vi "test Get Attribute as JSON Array2.vi"(11 "Test Case In":refnum<class "Test Config From Excel Table.lvclass">) -> (0 "error out":errorcluster, 3 "Test Case Out":refnum<class "Test Config From Excel Table.lvclass">)   [LabVIEW 2020, in "Test Config From Excel Table.lvclass"]
uses:
  Test Config From Excel Table.lvclass
  Test Config From Excel Table.lvclass/Test Config From Excel Table.ctl
  <vilib>/JDP Science/JSONtext/JSONtext.lvlib
  <vilib>/Astemes/LUnit/Test Case.lvclass
  Open-Xml-LabVIEW/Source/Open Xml.lvlib
  Source/Config from Excel Table/Config from Excel Table.lvclass
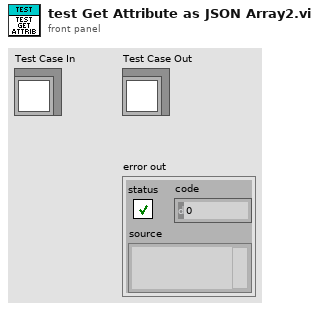
[diagram p1: front panel]
types:
  T1 = cluster{"Sheet Name":string, "Name":string, "Display Name":string, "Range or Cell Address":string}
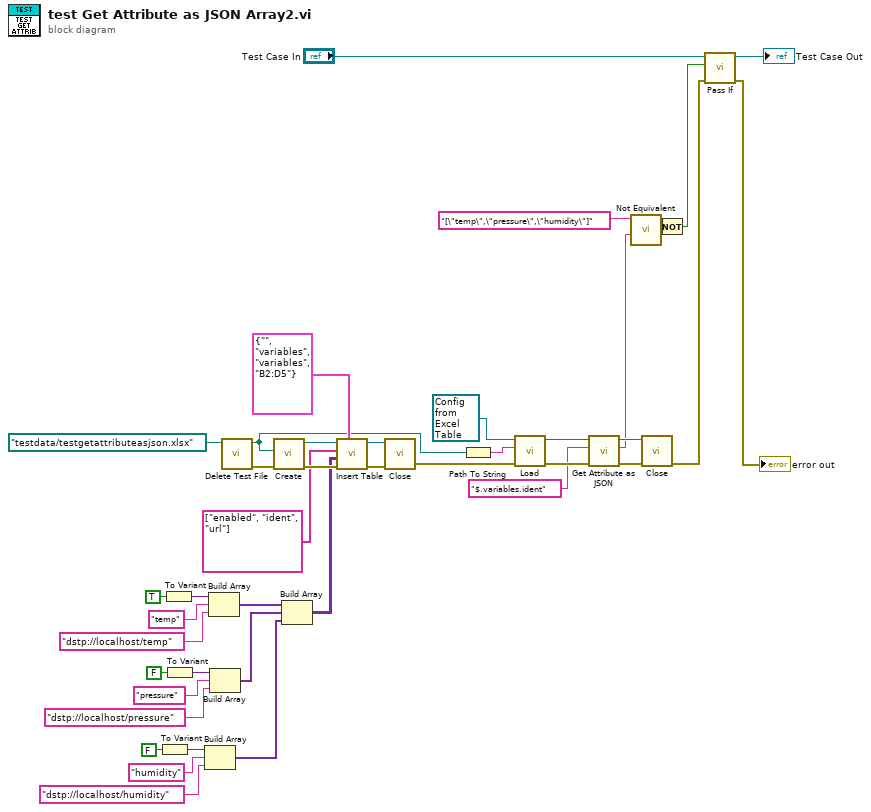
[diagram p0: block diagram]
diagram:
  n1 = To Variant(anything=FALSE) -> (Variant=w15:variant)
  n2 = To Variant(anything=TRUE) -> (Variant=w24:variant)
  n3 = To Variant(anything=FALSE) -> (Variant=w18:variant)
  n4 = Build Array(w15, "humidity", "dstp://localhost/humidity") -> (w11:variant[])
  n5 = Build Array(w24, "temp", "dstp://localhost/temp") -> (w21:variant[])
  n6 = Build Array(w18, "pressure", "dstp://localhost/pressure") -> (w12:variant[])
  n7 = call "Delete Test File.vi"("name or relative path"=path "testdata/testgetattributeasjson.xlsx") -> ("error out"=w29:errorcluster, "deleted path"=w3:path)  [unwired: 9 in]
  n8 = call "Create.vi"("error in"=w29, "Path"=w3) -> ("error out"=w28:errorcluster, "SpreadsheetDoc"=w9:refnum<k24>)  [unwired: 8 in]
  n9 = Build Array(w21, w12, w11) -> (w10:variant[][])
  n10 = call "Insert Table.vi"("Location"=T1 {"Sheet Name"="", "Name"="variables", "Display Name"="variables", "Range or Cell Address"="B2:D5"}, "error in"=w28, "Cell Values"=w10, "Header Names"=string[] ["enabled", "ident", "url"], "SpreadsheetDoc in"=w9) -> ("error out"=w8:errorcluster, "SpreadsheetDoc out"=w7:refnum<k24>)  [unwired: 5 in]
  n11 = call "Close.vi"("error in"=w8, "SpreadsheetDoc"=w7) -> ("error out"=w6:errorcluster)  [unwired: 9 in]
  n12 = Path To String(path=w3) -> (string=w38:string)
  n13 = call-dynamic "Load.vi"("error in"=w6, "Source"=w38, "Config from Excel Table in"=refnum<class "Config from Excel Table.lvclass"> refnum ("Config from EXCEL Table.lvclass")) -> ("error out"=w35:errorcluster, "Config from Excel Table out"=w36:refnum<class "Config from Excel Table.lvclass">)  [unwired: 7 in]
  n14 = call-dynamic "Get Attribute as JSON.vi"("error in"=w35, "Attribute"="$.variables.ident", "Config from Excel Table in"=w36) -> ("error out"=w33:errorcluster, "<JSON>"=w2:string, "Config from Excel Table out"=w32:refnum<class "Config from Excel Table.lvclass">)  [unwired: 6 in]
  n15 = call <vilib>:"Not Equivalent.vi"("Other JSON"=w2, "JSON"="[\"temp\",\"pressure\",\"humidity\"]" ("<JSON>")) -> ("Not Equivalent"=w31:bool)  [unwired: 8 in]
  n16 = call-dynamic "Close.vi"("error in"=w33, "Config from Excel Table in"=w32) -> ("error out"=w37:errorcluster)  [unwired: 8 in, 1 out]
  n17 = Not(x=w31) -> (.not. x?=w30:bool)
  n18 = call <vilib>:"Pass If.vi"("error in (no error)"=w37, "Pass?"=w30, "LUnit Test Case In"="Test Case In") -> ("error out"=→"error out":errorcluster, "LUnit Test Case Out"=→"Test Case Out":refnum<class "Test Config From Excel Table.lvclass">)  [unwired: 7 in]
